vi "Main.vi"(8 "error in (no error)":errorcluster, 11 "TemplateBase in":refnum<class "Cobolt.lvclass">) -> (0 "error out":errorcluster, 3 "component":refnum<class "Cobolt.lvclass">)   [LabVIEW 2012, in "Cobolt.lvclass"]
doc: "Main VI of the component."
uses:
  Cobolt.lvclass
  <vilib>/Distrio/Murmex/Murmex/command_enum.ctl
  laser lines.ctl
  Cobolt.lvclass/Cobolt.ctl
  <vilib>/Distrio/Murmex/InitialiseMessage/InitialiseMessage.lvclass
  <vilib>/Distrio/Murmex/ConfigureMessage/ConfigureMessage.lvclass
  <vilib>/Distrio/Murmex/GenericMessage/GenericMessage.lvclass
  <vilib>/Distrio/Murmex/TerminateMessage/TerminateMessage.lvclass
  <vilib>/Distrio/Murmex/Murmex/update_cluster.ctl
  <vilib>/Distrio/Murmex/Murmex/Set configure at initialise.vi
  <vilib>/Distrio/Murmex/Murmex/Set log reference.vi
  <vilib>/Distrio/Murmex/Murmex/Set VI reference.vi
  <vilib>/Distrio/Murmex/Murmex/Get ID.vi
  <vilib>/Distrio/Murmex/Message/Add or replace parameter.vi
  <vilib>/Distrio/Murmex/Murmex/Murmex.lvclass
  <vilib>/Distrio/Murmex/Message/Message.lvclass
panel:
  in  "button::configure":bool
  in  "button:quit":bool
  in  "Tab Control":enum32{"Main", "Debug COM", "Debug Murmex"}(tab)
  in  "Power":dbl[unit]=0.05 min=0.0 max=0.05 step=0.001 format="%#_1f"
  in  "VISA command":string(combo)
  out "Error":bool
  out "Lock":bool
  out "Laser":bool
  out "Power":bool
  in  "button::Shutter":bool
  in  "button::clear faults":bool
  in  "button::apply":bool
  out "Laser line":T1=9 items=["405nm"=4, "445nm"=6, "491nm"=8, "515nm"=9, "561nm"=10]
  out "Read  from COM":string
  in  "button::set key switch":bool
  out "Error Message":string
  out "Operating mode":string
  out "Keyswitch":bool
  out "Autostart":bool
  out "Response OK":bool
  in  "button::restart laser":bool
  out "log":string
  in  "ID":string
  in  "Generic command":string
  in  "button:send command":bool
  in  "command":T2
  out "terminate?":bool
  # "LEDs"
  # "Parameters"
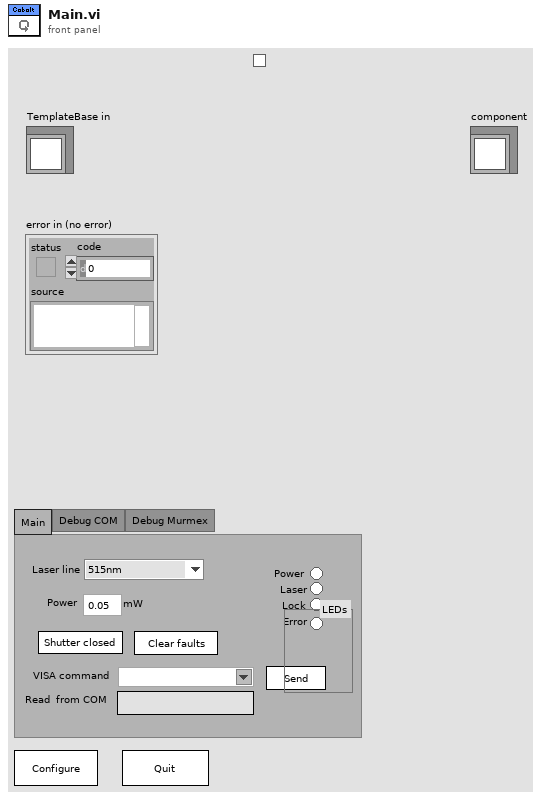
[diagram p1: front panel]
types:
  T1 = typedef "Cobolt.lvclass/laser lines.ctl" = u16
  T2 = typedef "Murmex.lvlib/Murmex.lvclass/command_enum.ctl" = enum16{"null", "initialise", "reset", "terminate", "acknowledge", "update", "inspect", "inform", "proceed", "start", "stop", "fetch", "configure", "generic"}
  T3 = enum8{"Enabled", "Disabled", "Disabled and Grayed Out"}
  T4 = typedef "Murmex.lvlib/Murmex.lvclass/update_cluster.ctl" = cluster{"target ID":string, "key chains":string[], "values":variant[]}
  T5 = typedef "Murmex.lvclass/command_enum.ctl" = enum16{"null", "initialise", "reset", "terminate", "acknowledge", "update", "inspect", "inform", "proceed", "start", "stop", "fetch", "configure", "generic"}
  T6 = typedef "Murmex.lvclass/Event type enumerations.ctl" = enum16{"before", "after"}
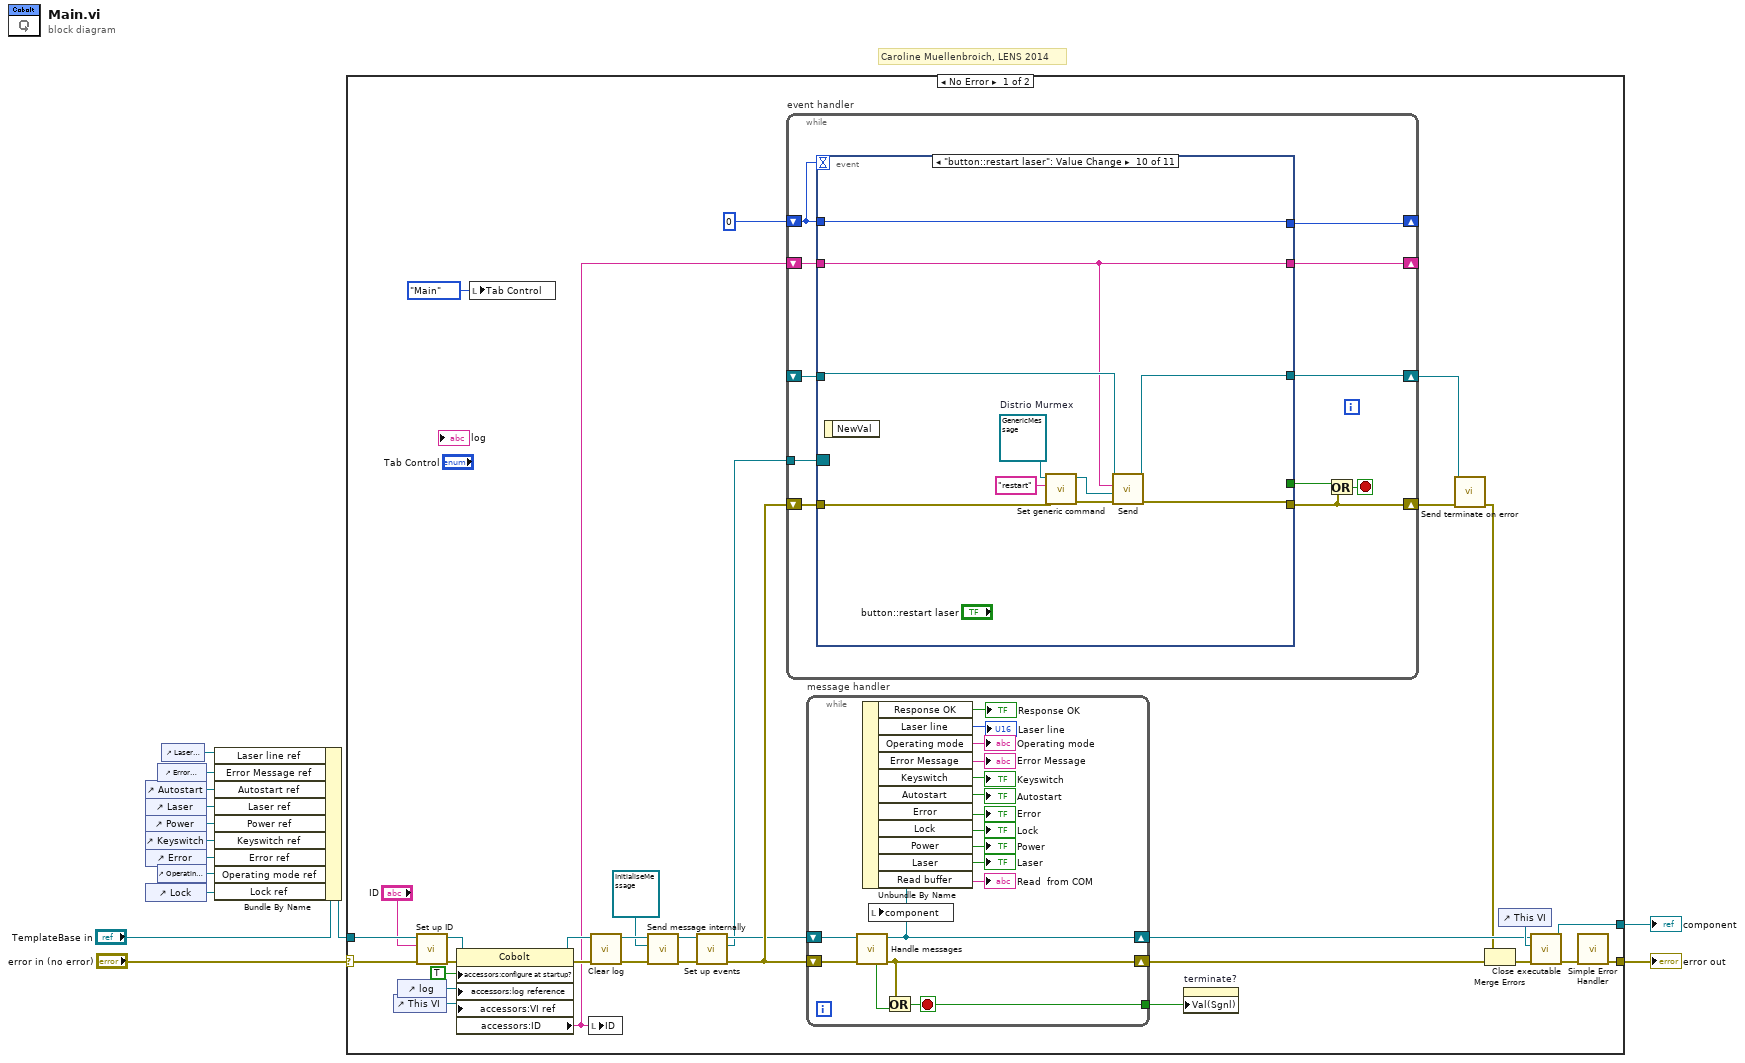
[diagram p0: block diagram]
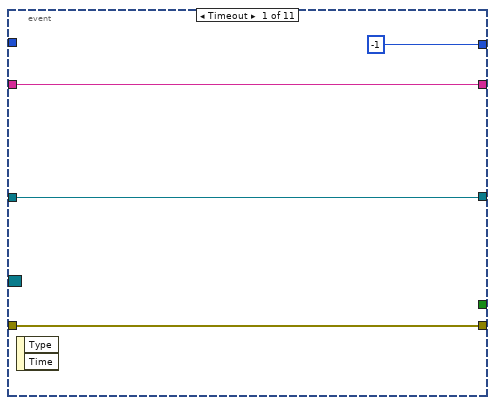
[diagram p2: hidden frame]
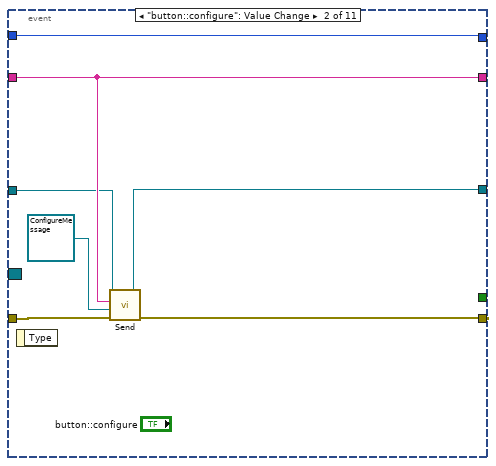
[diagram p3: hidden frame]
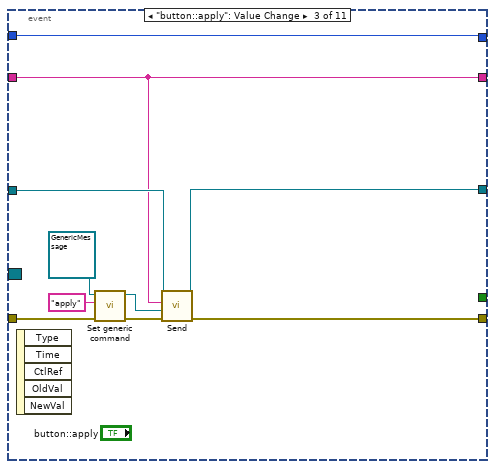
[diagram p4: hidden frame]
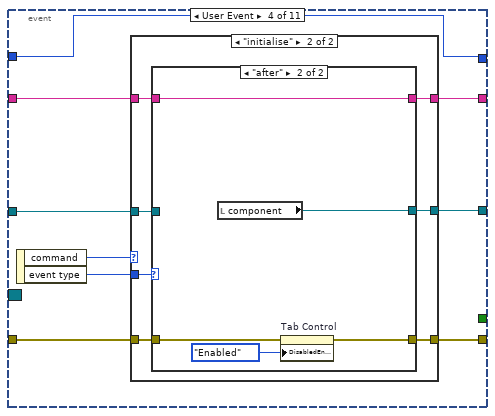
[diagram p5: hidden frame]
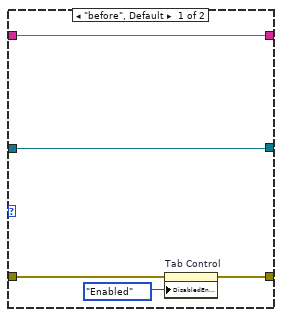
[diagram p7: hidden frame]
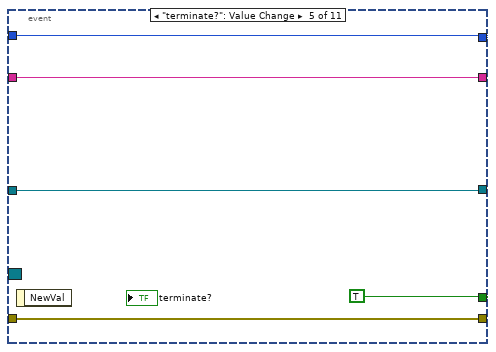
[diagram p8: hidden frame]
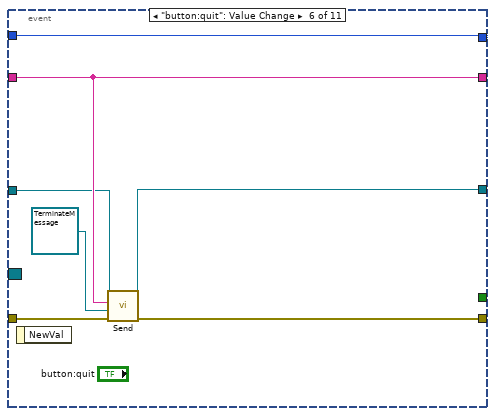
[diagram p9: hidden frame]
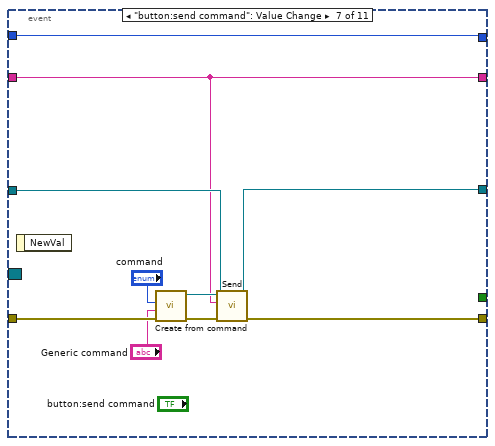
[diagram p10: hidden frame]
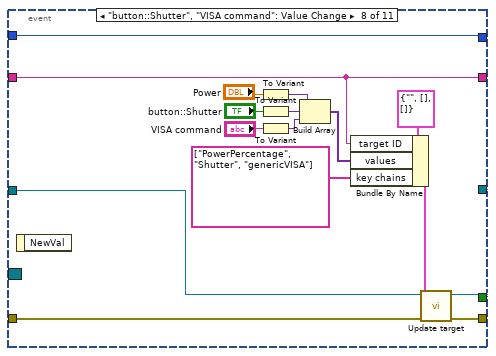
[diagram p11: hidden frame]
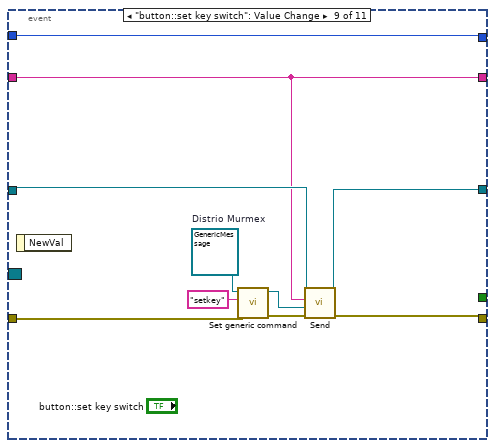
[diagram p12: hidden frame]
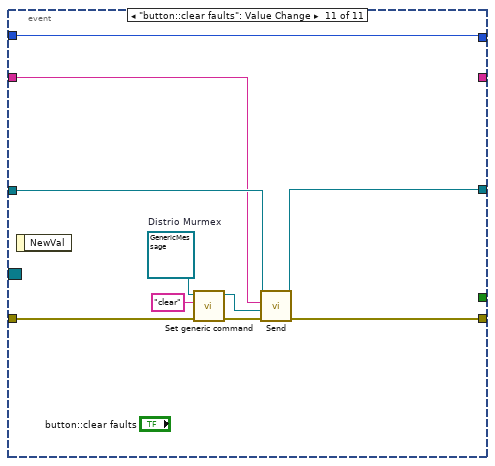
[diagram p13: hidden frame]
diagram:
  # "Caroline Muellenbroich, LENS 2014"
  n1 = control-ref of="Autostart"() -> (w3:refnum<vi>)
  n2 = control-ref of="Laser"() -> (w4:refnum<vi>)
  n3 = control-ref of="Power"() -> (w5:refnum<vi>)
  n4 = control-ref of="Keyswitch"() -> (w6:refnum<vi>)
  n5 = control-ref of="Error"() -> (w7:refnum<vi>)
  n6 = control-ref of="Lock"() -> (w9:refnum<vi>)
  n7 = control-ref of="Error Message"() -> (w2:refnum<vi>)
  n8 = control-ref of="Operating mode"() -> (w8:refnum<vi>)
  n9 = control-ref of="Laser line"() -> (w1:refnum<vi>)
  n10 = Bundle By Name(cluster="TemplateBase in", "Laser line ref"=w1, "Error Message ref"=w2, "Autostart ref"=w3, "Laser ref"=w4, "Power ref"=w5, "Keyswitch ref"=w6, "Error ref"=w7, "Operating mode ref"=w8, "Lock ref"=w9) -> (w10:refnum<class "Cobolt.lvclass">)
  n11 = case shown="No Error" "error in (no error)" {
    selector: "error in (no error)" -> [w34 w193]
    tunnel: [w27 w194] -> w14
    tunnel: w10 -> [w36 w194]
    tunnel: [w29 w193] -> w13
    frame No Error {
      n12 = control-ref of="This VI"() -> (w43:refnum<vi>)
      n13 = control-ref of="log"() -> (w44:refnum<vi>)
      n14 = call <vilib>:"Set up ID.vi"("error in (no error)"=w34, "component ID"="ID", "MurmexBase in"=w36) -> ("error out"=w37:errorcluster, "MurmexBase out"=w35:refnum<class "Cobolt.lvclass">)  [unwired: 6 in, 1 out]
      n15 = property class="Cobolt"(reference=w35, error in=w37, "accessors:configure at startup?"=TRUE ("configure at startup?"), "accessors:log reference"=w44, "accessors:VI ref"=w43) -> (reference out=w46:refnum<class "Cobolt.lvclass">, error out=w41:errorcluster, "accessors:ID"=w16:string)
      n16 = local write "Tab Control"(enum32{"Main", "Debug COM", "Debug Murmex"}."Main" ("Tab Control")) -> ()
      n17 = local write "ID"(w16) -> ()
      n18 = call <vilib>:"Clear log.vi"("error in (no error)"=w41, "MurmexBase in"=w46) -> ("error out"=w40:errorcluster, "MurmexBase out"=w42:refnum<class "Cobolt.lvclass">)  [unwired: 8 in]
      n19 = call <vilib>:"Send message internally.vi"("error in (no error)"=w40, "Message"=refnum<class "InitialiseMessage.lvclass"> refnum, "Murmex in"=w42) -> ("error out"=w38:errorcluster, "Murmex out"=w26:refnum<class "Cobolt.lvclass">)  [unwired: 7 in]
      n20 = call <vilib>:"Set up events.vi"("error in (no error)"=w38, "MurmexBase in"=w26) -> ("error out"=w33:errorcluster, "Event Registration Refnum"=w21:refnum<event-registration>, "MurmexBase out"=w25:refnum<class "Cobolt.lvclass">)  [unwired: 7 in]
      n21 = while "event handler" {
        shift-right: [w56] -> w23
        shift-left: w33 -> [w57]
        shift-right: [w53] -> _
        shift-left: 0 -> [w47]
        tunnel: w21 -> [w52]
        shift-right: [w50] -> _
        shift-left: w16 -> [w51]
        shift-right: [w49] -> w19
        shift-left: _ -> [w48]
        stop <- w54 stop-if-true
        n22 = event shown="[9] \"button::restart laser\": Value Change" {
          selector: w52 -> [_ _ _ _ _ _ _ _ _ _ _]
          dyn-events: _ -> [_ _ _ _ _ _ _ _ _ _ _]
          timeout: w47 -> [_ _ _ _ _ _ _ _ _ _ _]
          tunnel: w57 -> [w61 w68 w75 w87 w112 w118 w129 w138 w151 w161 w171]
          tunnel: [w61 w63 w74 w79 w112 w119 w127 w136 w150 w160 w170] -> w56
          tunnel: [_ _ _ _ TRUE _ _ _ _ _ _] -> w55
          tunnel: w47 -> [_ w64 w70 w80 w110 w114 w121 w133 w147 w157 w166]
          tunnel: [-1 w64 w70 w80 w110 w114 w121 w133 w147 w157 w166] -> w53
          tunnel: w51 -> [w59 w67 w71 w82 w109 w117 w122 w137 w146 w156 w167]
          tunnel: [w59 w67 w71 w81 w109 w117 w122 w137 w146 w156 _] -> w50
          tunnel: [w58 w65 w72 w84 w108 w115 w124 w134 w148 w158 w168] -> w49
          tunnel: w48 -> [w58 w66 w73 w83 w108 w116 w125 w135 w149 w159 w169]
          event Timeout {
            n23 = event-data() -> ()  [unwired: 1 in, 2 out]
          }
          event "button::configure": Value Change {
            n24 = event-data() -> ()  [unwired: 1 in, 1 out]
            n25 = call <vilib>:"Send.vi"("error in (no error)"=w68, "Message"=refnum<class "ConfigureMessage.lvclass"> refnum ("Distrio Murmex"), "recipient"=w67, "Murmex in"=w66) -> ("error out"=w63:errorcluster, "Murmex out"=w65:refnum<class "Murmex.lvclass">)  [unwired: 6 in]
          }
          event "button::apply": Value Change {
            n26 = event-data() -> ()  [unwired: 1 in, 5 out]
            n27 = call <vilib>:"Set generic command.vi"("error in (no error)"=w75, "generic command"="apply", "GenericMessage in"=refnum<class "GenericMessage.lvclass"> refnum ("Distrio Murmex")) -> ("error out"=w77:errorcluster, "GenericMessage out"=w76:refnum<class "GenericMessage.lvclass">)  [unwired: 7 in]
            n28 = call <vilib>:"Send.vi"("error in (no error)"=w77, "Message"=w76, "recipient"=w71, "Murmex in"=w73) -> ("error out"=w74:errorcluster, "Murmex out"=w72:refnum<class "Murmex.lvclass">)  [unwired: 6 in]
          }
          event User Event {
            n29 = event-data() -> ("command"=w86:T5, "event type"=w85:T6)  [unwired: 1 in]
            n30 = case shown="\"initialise\"" w86 {
              tunnel: w85 -> [_ w97]
              tunnel: w87 -> [w90 w96]
              tunnel: [w90 w95] -> w79
              tunnel: [w89 w94] -> w84
              tunnel: w83 -> [w89 w93]
              tunnel: w82 -> [w88 w92]
              tunnel: [w88 w91] -> w81
              frame "null", Default {
              }
              frame "initialise" {
                n31 = case shown="\"after\"" w97 {
                  tunnel: [w101 w105] -> w95
                  tunnel: w96 -> [w102 w106]
                  tunnel: [w99 w107] -> w94
                  tunnel: w93 -> [w99 _]
                  tunnel: w92 -> [w98 w103]
                  tunnel: [w98 w103] -> w91
                  frame "before", Default {
                    n32 = property on="Tab Control" class="TabCtl (strict)"(error in=w102, "DisabledEnum"=T3."Enabled" ("Disabled")) -> (error out=w101:errorcluster)  [unwired: 1 in, 1 out]
                  }
                  frame "after" {
                    n33 = local read "component"() -> (w107:refnum<class "Cobolt.lvclass">)
                    n34 = property on="Tab Control" class="TabCtl (strict)"(error in=w106, "DisabledEnum"=T3."Enabled" ("Disabled")) -> (error out=w105:errorcluster)  [unwired: 1 in, 1 out]
                  }
                }
              }
            }
          }
          event "terminate?": Value Change {
            n35 = event-data() -> ()  [unwired: 1 in, 1 out]
          }
          event "button:quit": Value Change {
            n36 = event-data() -> ()  [unwired: 1 in, 1 out]
            n37 = call <vilib>:"Send.vi"("error in (no error)"=w118, "Message"=refnum<class "TerminateMessage.lvclass"> refnum ("Distrio Murmex 1.1:TerminateMessage"), "recipient"=w117, "Murmex in"=w116) -> ("error out"=w119:errorcluster, "Murmex out"=w115:refnum<class "Murmex.lvclass">)  [unwired: 6 in]
          }
          event "button:send command": Value Change {
            n38 = event-data() -> ()  [unwired: 1 in, 1 out]
            n39 = call <vilib>:"Create from command.vi"("error in (no error)"=w129, "generic command"="Generic command", "command"="command") -> ("error out"=w123:errorcluster, "Message out"=w128:refnum<class "Message.lvclass">)  [unwired: 7 in]
            n40 = call <vilib>:"Send.vi"("error in (no error)"=w123, "Message"=w128, "recipient"=w122, "Murmex in"=w125) -> ("error out"=w127:errorcluster, "Murmex out"=w124:refnum<class "Murmex.lvclass">)  [unwired: 6 in]
          }
          event "button::Shutter", "VISA command": Value Change {
            n41 = event-data() -> ()  [unwired: 1 in, 1 out]
            n42 = To Variant(anything="Power") -> (Variant=w145:variant)
            n43 = To Variant(anything="button::Shutter") -> (Variant=w144:variant)
            n44 = To Variant(anything="VISA command") -> (Variant=w132:variant)
            n45 = Build Array(w145, w144, w132) -> (w142:variant[])
            n46 = Bundle By Name(cluster=T4 {"target ID"="", "key chains"=[], "values"=[]} ("update cluster"), "target ID"=w137, "values"=w142, "key chains"=string[] ["PowerPercentage", "Shutter", "genericVISA"]) -> (w139:T4)
            n47 = call <vilib>:"Update target.vi"("error in (no error)"=w138, "update cluster"=w139, "MurmexBase in"=w135) -> ("error out"=w136:errorcluster, "MurmexBase out"=w134:refnum<class "Murmex.lvclass">)  [unwired: 7 in]
          }
          event "button::set key switch": Value Change {
            w155 = refnum<class "GenericMessage.lvclass"> refnum  # Distrio Murmex
            n48 = event-data() -> ()  [unwired: 1 in, 1 out]
            n49 = call <vilib>:"Set generic command.vi"("error in (no error)"=w151, "generic command"="setkey", "GenericMessage in"=w155) -> ("error out"=w153:errorcluster, "GenericMessage out"=w154:refnum<class "GenericMessage.lvclass">)  [unwired: 7 in]
            n50 = call <vilib>:"Send.vi"("error in (no error)"=w153, "Message"=w154, "recipient"=w146, "Murmex in"=w149) -> ("error out"=w150:errorcluster, "Murmex out"=w148:refnum<class "Murmex.lvclass">)  [unwired: 6 in]
          }
          event "button::restart laser": Value Change {
            w165 = refnum<class "GenericMessage.lvclass"> refnum  # Distrio Murmex
            n51 = event-data() -> ()  [unwired: 1 in, 1 out]
            n52 = call <vilib>:"Set generic command.vi"("error in (no error)"=w161, "generic command"="restart", "GenericMessage in"=w165) -> ("error out"=w163:errorcluster, "GenericMessage out"=w164:refnum<class "GenericMessage.lvclass">)  [unwired: 7 in]
            n53 = call <vilib>:"Send.vi"("error in (no error)"=w163, "Message"=w164, "recipient"=w156, "Murmex in"=w159) -> ("error out"=w160:errorcluster, "Murmex out"=w158:refnum<class "Murmex.lvclass">)  [unwired: 6 in]
          }
          event "button::clear faults": Value Change {
            w172 = refnum<class "GenericMessage.lvclass"> refnum  # Distrio Murmex
            n54 = event-data() -> ()  [unwired: 1 in, 1 out]
            n55 = call <vilib>:"Set generic command.vi"("error in (no error)"=w171, "generic command"="clear", "GenericMessage in"=w172) -> ("error out"=w174:errorcluster, "GenericMessage out"=w173:refnum<class "GenericMessage.lvclass">)  [unwired: 7 in]
            n56 = call <vilib>:"Send.vi"("error in (no error)"=w174, "Message"=w173, "recipient"=w167, "Murmex in"=w169) -> ("error out"=w170:errorcluster, "Murmex out"=w168:refnum<class "Murmex.lvclass">)  [unwired: 6 in]
          }
        }
        n57 = Or(x=w55, y=w56) -> (x .or. y?=w54:bool)
      }
      n58 = while "message handler" {
        shift-right: [w179] -> w15
        shift-left: w33 -> [w192]
        shift-right: [w178] -> w28
        shift-left: w25 -> [w191]
        tunnel: [w189] -> w39
        stop <- w189 stop-if-true
        n59 = call <vilib>:"Handle messages.vi"("error in (no error)"=w192, "Murmex in"=w191) -> ("error out"=w179:errorcluster, "Murmex out"=w178:refnum<class "Cobolt.lvclass">, "terminated?"=w190:bool)  [unwired: 7 in]
        n60 = Unbundle By Name(w178) -> ("Response OK"=→"Response OK":bool, "Laser line"=→"Laser line":T1, "Operating mode"=→"Operating mode":string, "Error Message"=→"Error Message":string, "Keyswitch"=→"Keyswitch":bool, "Autostart"=→"Autostart":bool, "Error"=→"Error":bool, "Lock"=→"Lock":bool, "Power"=→"Power":bool, "Laser"=→"Laser":bool, "Read buffer"=→"Read  from COM":string)
        n61 = local write "component"(w178) -> ()
        n62 = Or(x=w179, y=w190) -> (x .or. y?=w189:bool)
      }
      n63 = property on="terminate?" class="Bool (strict)"("Val(Sgnl)"=w39) -> ()  [unwired: 2 in, 2 out]
      n64 = call <vilib>:"Send terminate on error.vi"("error in (no error)"=w23, "Murmex in"=w19) -> ("error out"=w24:errorcluster)  [unwired: 8 in, 1 out]
      n65 = Merge Errors(w24, w15) -> (w32:errorcluster)
      n66 = control-ref of="This VI"() -> (w30:refnum<vi>)
      n67 = call <vilib>:"Close executable.vi"("error in (no error)"=w32, "main VI ref (optional)"=w30, "MurmexBase in"=w28) -> ("error out"=w31:errorcluster, "MurmexBase out"=w27:refnum<class "Cobolt.lvclass">)  [unwired: 7 in]
      n68 = call <vilib>:"Simple Error Handler.vi"("error in (no error)"=w31) -> ("error out"=w29:errorcluster)  [unwired: 4 in, 4 out]
    }
    frame Error {
    }
  }
  "error out" <- w13
  "component" <- w14
